vi "DtCreateCtrUpDownChan.vi"(5 "Board Name":string, 7 "Counter Num":u32, 11 "error in (no error)":errorcluster) -> (4 "Task out":i32, 15 "error out":errorcluster)   [LabVIEW 2016]
doc: "Creates one or more virtual counter/timer channels that count digital pulses from an external signal that is connected to the counter/timer's clock input source. If the gate input signal of the counter/timer is high, the count is incremented. If the gate input signal of the counter/timer is low, the count is decremented.\n\nThis type of task is also known as up/down counting. To use this VI, your device must support up/down counting mode.\n\nOnce you have created a virtual counter/timer channel for an up/down counting task, you can start the task and read the count using the DtOLRead (Read Single Channel - Single Sample) VI."
uses:
  <userlib>/LV-Link3/DtLvLink.lvlib
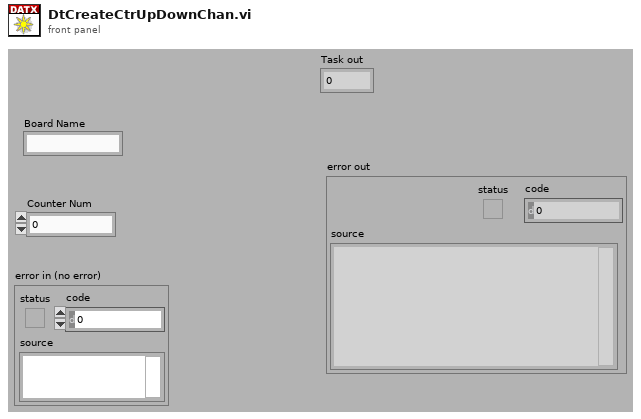
[diagram p1: front panel]
types:
  T1 = enum32{"AnalogInput", "AnalogOutput", "DigitalInput", "DigitalOutput", "Quadrature", "CounterTimer"}
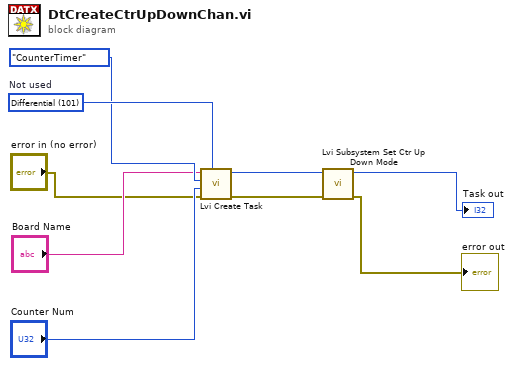
[diagram p0: block diagram]
diagram:
  w9 = 101 items=["SingleEnded"=100, "Differential"=101]  # Not used
  n1 = call <userlib>:"Lvi Create Task.vi"("SEorDiff"=w9, "error in (no error)"="error in (no error)", "SubSysIndex"="Counter Num", "ChanType"=T1."CounterTimer", "BoardName"="Board Name") -> ("error out"=w6:errorcluster, "TaskRef"=w7:i32)  [unwired: 4 in, 1 out]
  n2 = call <userlib>:"Lvi Subsystem Set Ctr Up Down Mode.vi"("error in (no error)"=w6, "TaskRef"=w7) -> ("error out"=→"error out":errorcluster, "TaskRef out"=→"Task out":i32)  [unwired: 7 in, 1 out]
